vi "GetTrendValue_from_metric_ID.vi"(7 "Input: trend id":string, 11 "TrendPoints":T1[](array[typedef])) -> (3 "Value":dbl)   [LabVIEW 2017]
uses:
  <vilib>/addons/InsightCM/MessageBus/Base/controls/TrendPoint.ctl
  <vilib>/addons/InsightCM/MessageBus/Base/controls/KeyValuePair.ctl
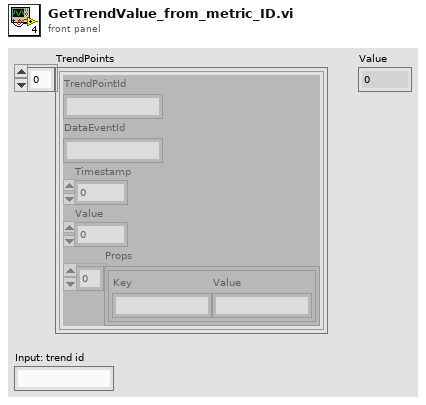
[diagram p1: front panel]
types:
  T1 = typedef "TrendPoint.ctl" = cluster{"TrendPointId":string, "DataEventId":string, "Timestamp":i64, "Value":dbl, "Props":T2[]}
  T2 = typedef "KeyValuePair.ctl" = cluster{"Key":string, "Value":string}
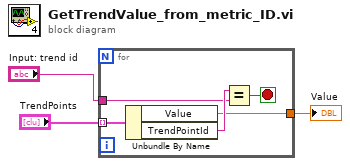
[diagram p0: block diagram]
diagram:
  n1 = for {
    tunnel: "TrendPoints" -> [w8] mode=indexing
    tunnel: "Input: trend id" -> [w6]
    tunnel: [w4] -> w2
    stop <- w5 stop-if-true
    n2 = Unbundle By Name(w8) -> ("Value"=w4:dbl, "TrendPointId"=w7:string)
    n3 = Equal?(x=w7, y=w6) -> (x = y?=w5:bool)
  }
  "Value" <- w2
